vi "Find Log Record.vi"(8 "Error In":errorcluster) -> (0 "Error Out":errorcluster, 2 "Names":string[](array[string]), 3 "Module List":refnum<class "Process Object.lvclass">[](array[class]))   [LabVIEW 2020]
uses:
  Log Record.lvclass
  C:/GitHub/LabActor/Process Object/Process Object.lvclass
  C:/GitHub/LabActor/Worker/Worker.lvclass
  C:/GitHub/LabActor/Template Module/Template Module.lvclass
  C:/Program Files/National Instruments/LabVIEW 2020/vi.lib/ActorFramework/Actor/Actor.lvclass
  C:/GitHub/LabActor/Post-Processors/Log Record/Log Record.lvclass
  Process Object/Process Object.lvclass
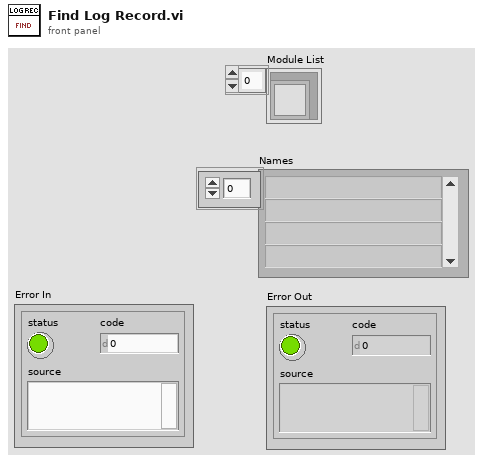
[diagram p1: front panel]
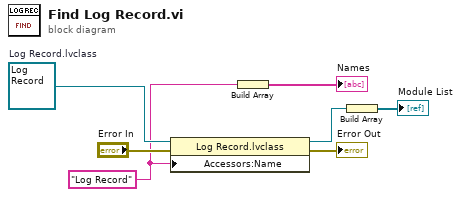
[diagram p0: block diagram]
diagram:
  w6 = refnum<class "Log Record.lvclass"> refnum  # Log Record.lvclass
  w3 = "Log Record" ("Name")
  n1 = property class="Log Record.lvclass"(reference=w6, error in="Error In", "Accessors:Name"=w3) -> (reference out=w2:refnum<class "Log Record.lvclass">, error out=→"Error Out":errorcluster)
  n2 = Build Array(w3) -> (→"Names":string[])
  n3 = Build Array(w2) -> (→"Module List":refnum<class "Log Record.lvclass">[])
